vi "002FH_氯化物_第一点校正指令写入.vi"(8 "error in (no error)":errorcluster caption="错误输入（无错误）", 10 "数值":u16=17 format="%xH", 11 "MB session in":refnum<class "MB_Master.lvclass">) -> (0 "error out":errorcluster caption="错误输出", 3 "MB session out":refnum<class "MB_Master.lvclass">)   [LabVIEW 2016, in "斯坦道多参数.lvlib"]
uses:
  <vilib>/Plasmionique/MB Master/MB Master.lvlib
  <vilib>/Plasmionique/MB Master/MB_Master/MB_Master.lvclass
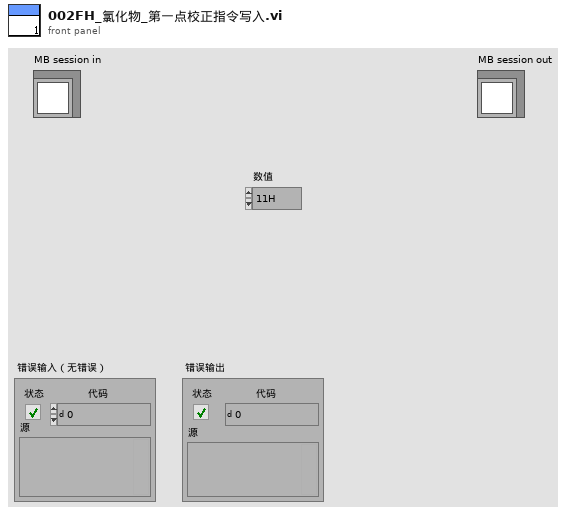
[diagram p1: front panel]
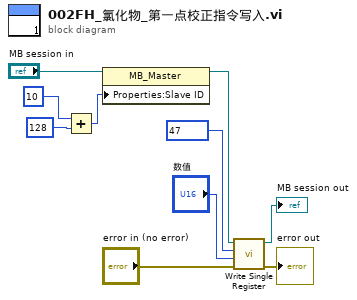
[diagram p0: block diagram]
diagram:
  n1 = Add(x=u16 10 ("y"), y=u16 128) -> (x+y=w6:u16)
  n2 = property class="MB_Master"(reference="MB session in", "Properties:Slave ID"=w6) -> (reference out=w4:refnum<class "MB_Master.lvclass">)  [unwired: 1 in, 1 out]
  n3 = call <vilib>:"Write Single Register.vi"("error in (no error)"="error in (no error)", "value"="数值", "address"=u16 47 ("starting address"), "MB session in"=w4) -> ("error out"=→"error out":errorcluster, "MB session out"=→"MB session out":refnum<class "MB_Master.lvclass">)  [unwired: 6 in]
